vi "file_check_label.vi"(4 "Loop Data Labels":string[][](array[string])=[["Vap Mass Flow", "Liq Mass Flow", "DP", "Liq Tank P", "LiqTank T", "Sep P", "SepT", "Liq In P", "Liq In T", "Vap Tank P", "Vap Tank T", "Dev Section P", "Dev Section T", "Up TS P", "Up TS T", "Low TS P", "Low TS T", "Cond Top T", "Evap Top T", "Cond Bot T", "Evap Bot T", "Win 3-4 P", "Top Heat T", "Bot Heat T"]], 5 "index":dbl) -> (0 "error out":errorcluster, 1 "dup path":path)   [LabVIEW 2017]
uses:
  <vilib>/Utility/sysdir.llb/System Directory Type.ctl
  <vilib>/Utility/file.llb/Write Delimited Spreadsheet (string).vi
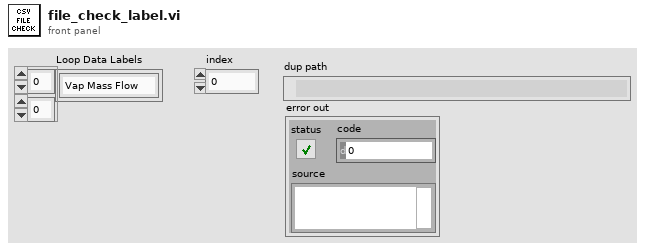
[diagram p1: front panel]
types:
  T1 = typedef "System Directory Type.ctl" = i32
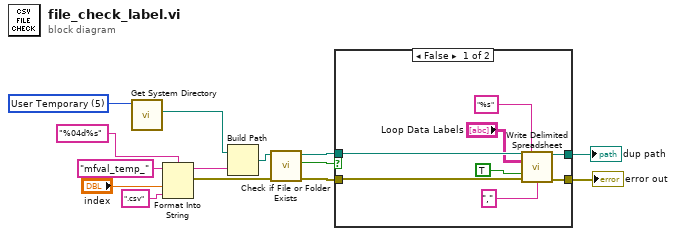
[diagram p0: block diagram]
diagram:
  w3 = T1 5 items=["User Home"=0, "User Desktop"=1, "User Documents"=2, "User Application Data"=3, "User Preferences"=4, "User Temporary"=5, "Public Documents"=6, "Public Application Data"=7, "Public Preferences"=8, "Public Cache"=13, "System Core Libraries"=9, "System Installed Libraries"=10, "Application Files"=11, "Boot Volume Root"=12] ("system directory type")
  n1 = call <vilib>:"Get System Directory.vi"("system directory type"=w3) -> ("system directory"=w2:path)  [unwired: 10 in]
  n2 = Format Into String(format string="%04d%s", initial string="mfval_temp_", "index", ".csv") -> (resulting string=w14:string, error out=w12:errorcluster)  [unwired: 1 in]
  n3 = Build Path(base path=w2, name or relative path=w14) -> (appended path=w13:path)
  n4 = call <vilib>:"Check if File or Folder Exists.vi"("error in (no error)"=w12, "path"=w13) -> ("error out"=w9:errorcluster, "file or folder exists?"=w11:bool, "dup path"=w10:path)  [unwired: 7 in]
  n5 = case shown="False" w11 {
    tunnel: [w22 w24] -> w5
    tunnel: w10 -> [w18 w24]
    tunnel: [w21 w23] -> w4
    tunnel: w9 -> [w17 w23]
    frame False {
      n6 = call-poly <vilib>:"Write Delimited Spreadsheet.vi"("file path (dialog if empty)"=w18, "format (%s)"="%s", "2D data"="Loop Data Labels", "append to file? (new file:F)"=TRUE, "error in (no error)"=w17, "delimiter (\\t)"="," ("delimiter (\\t)")) -> ("new file path (Not A Path if cancelled)"=w22:path, "error out"=w21:errorcluster)  [unwired: 8 in]
    }
    frame True {
    }
  }
  "dup path" <- w5
  "error out" <- w4
